vi "Destroy.vi"(8 "error in (no error)":errorcluster, 11 "WebBrowser_Mgmt in":refnum<class "WebBrowser_Mgmt.lvclass">) -> (0 "error out":errorcluster, 3 "WebBrowser_Mgmt out":refnum<class "WebBrowser_Mgmt.lvclass">)   [LabVIEW 2016, in "WebBrowser_Mgmt.lvclass"]
uses:
  WebBrowser_Mgmt.lvclass
  WebBrowser_Mgmt.lvclass/WebBrowser_Mgmt.ctl
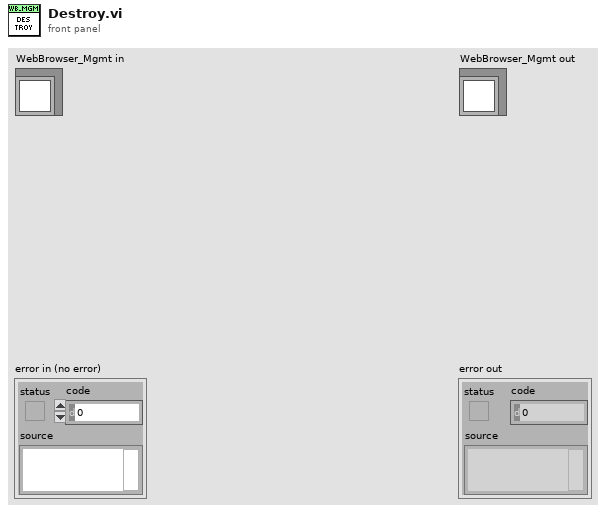
[diagram p1: front panel]
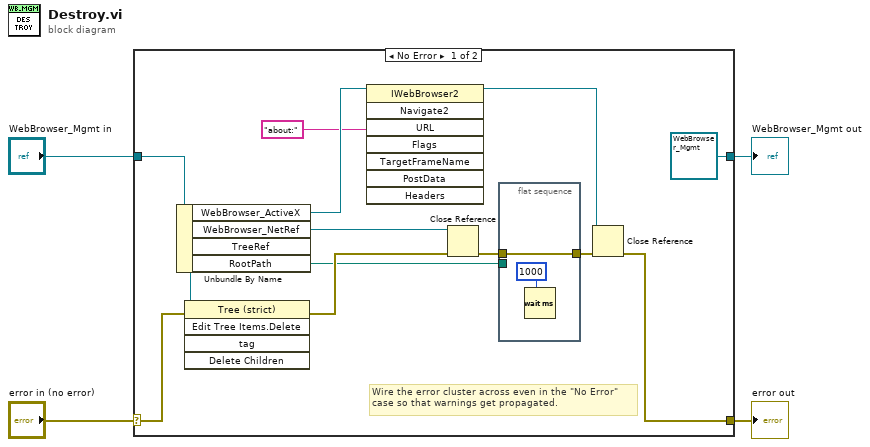
[diagram p0: block diagram]
diagram:
  n1 = case shown="No Error" "error in (no error)" {
    selector: "error in (no error)" -> [w7 w21]
    tunnel: [w14 w21] -> w3
    tunnel: [refnum<class "WebBrowser_Mgmt.lvclass"> refnum ("WebBrowser_Mgmt in") w20] -> w1
    tunnel: "WebBrowser_Mgmt in" -> [w17 w20]
    frame No Error {
      # "Wire the error cluster across even in the \"No Error\"\ncase so that warnings get propagated."
      n2 = Unbundle By Name(w17) -> ("WebBrowser_ActiveX"=w13:refnum<k7>, "WebBrowser_NetRef"=w16:refnum<k24>, "TreeRef"=w8:refnum<vi>, "RootPath"=w5:path)
      n3 = invoke class="Tree (strict)" method="Edit Tree Items.Delete"(reference=w8, error in=w7) -> (error out=w6:errorcluster)  [unwired: 3 in, 4 out]
      n4 = invoke class="IWebBrowser2" method="Navigate2"(reference=w13, "URL"="about:") -> (reference out=w12:refnum<k7>)  [unwired: 6 in, 7 out]
      n5 = Close Reference(reference=w16, error in (no error)=w6) -> (error out=w10:errorcluster)
      n6 = flat-sequence {
        tunnel: w10 -> [w19]
        tunnel: [w19] -> w9
        tunnel: w5 -> [_]
        frame #0 {
          n7 = Wait (ms)(milliseconds to wait=u32 1000) -> ()  [unwired: 1 out]
        }
      }
      n8 = Close Reference(reference=w12, error in (no error)=w9) -> (error out=w14:errorcluster)
    }
    frame Error {
    }
  }
  "error out" <- w3
  "WebBrowser_Mgmt out" <- w1
